vi "仁科告警状态解析.vi"(11 "告警状态输入":u16[](array[numeric])) -> (3 "告警状态":T1)   [LabVIEW 2016, in "环境动力监测库.lvlib" / "空调库.lvlib"]
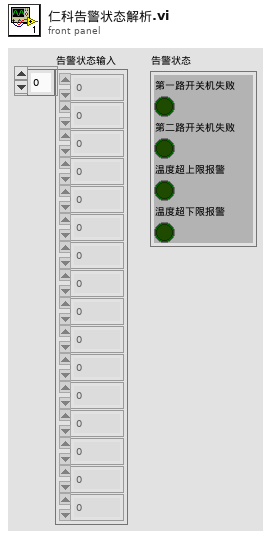
[diagram p1: front panel]
types:
  T1 = cluster{"第一路开关机失败":bool, "第二路开关机失败":bool, "温度超上限报警":bool, "温度超下限报警":bool}
  T2 = cluster{"[0]":bool, "[1]":bool, "[2]":bool, "[3]":bool}
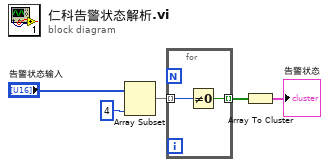
[diagram p0: block diagram]
diagram:
  n1 = Array Subset(array="告警状态输入", length=4 ("长度")) -> (w3:u16[])  [unwired: 1 in]
  n2 = for {
    tunnel: w3 -> [w7] mode=indexing
    tunnel: [w6] -> w2 mode=indexing
    n3 = Not Equal To 0?(x=w7) -> (x != 0?=w6:bool)
  }
  n4 = Array To Cluster(array=w2) -> (cluster=→"告警状态":T2)
